vi "sub_Boolean_Property.vi"() -> ()   [LabVIEW 2023]
panel:
  in  "Array":refnum<vi>[](array[refnum])
  in  "active":bool
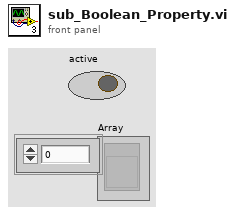
[diagram p1: front panel]
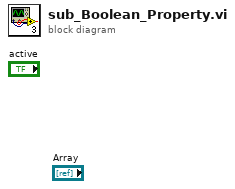
[diagram p0: block diagram]
diagram:
